vi "Close Connection.vi"(8 "error in (no error)":errorcluster, 11 "TCP Connection in":refnum<class "TCP Connection.lvclass">) -> (0 "error out":errorcluster, 3 "TCP Connection out":refnum<class "TCP Connection.lvclass">)   [LabVIEW 2012, in "TCP Classes.lvlib" / "TCP Connection.lvclass"]
uses:
  TCP Connection.lvclass
  TCP Connection.lvclass/TCP Connection.ctl
  <userlib>/STM/TCP/stm_TCP Connection Info.ctl
  <userlib>/STM/_SubVIs/stm_MetaDataElement.ctl
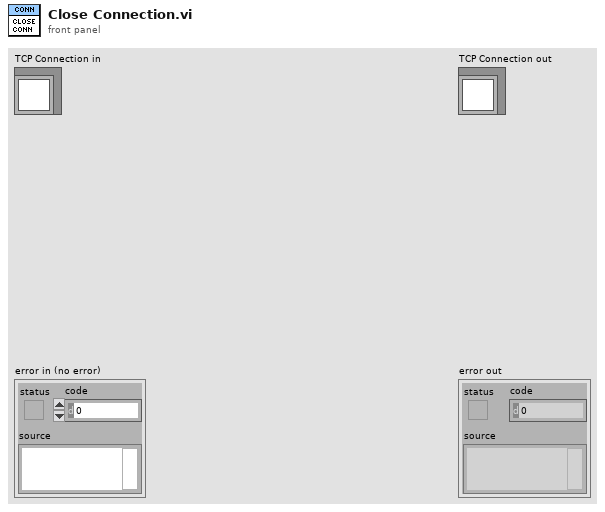
[diagram p1: front panel]
types:
  T1 = typedef "stm_TCP Connection Info.ctl" = cluster{"connection ID":refnum<k5>, "Meta data":T2[]}
  T2 = typedef "stm_MetaDataElement.ctl" = string
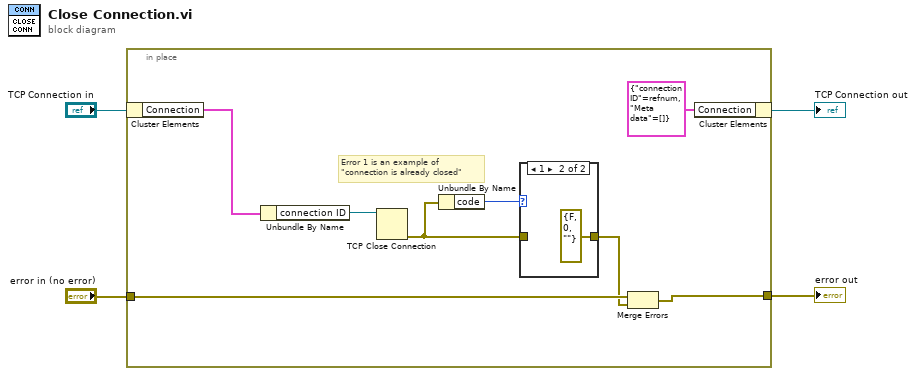
[diagram p0: block diagram]
diagram:
  n1 = in-place {
    in-place-border: "error in (no error)" -> [w10]
    in-place-border: [w8] -> w3
    # "Error 1 is an example of\n\"connection is already closed\""
    n2 = in-place-cluster #1("TCP Connection in") -> ("Connection"=w6:T1)
    n3 = Unbundle By Name(w6) -> ("connection ID"=w5:refnum<k5>)
    n4 = TCP Close Connection(connection ID=w5) -> (error out=w11:errorcluster)  [unwired: 2 in, 1 out]
    n5 = Unbundle By Name(w11) -> ("code"=w12:i32)
    n6 = case shown="1" w12 {
      tunnel: w11 -> [w13 _]
      tunnel: [w13 errorcluster {"status"=FALSE, "code"=0, "source"=""} ("error out")] -> w9
      frame Default {
      }
      frame 1 {
      }
    }
    n7 = Merge Errors(w10, w9) -> (w8:errorcluster)
    n8 = in-place-cluster #1("Connection"=T1 {"connection ID"=refnum, "Meta data"=[]}) -> (→"TCP Connection out":refnum<class "TCP Connection.lvclass">)
  }
  "error out" <- w3
